vi "GlobalVariables.vi"() -> ()   [LabVIEW 2020]
panel:
  in  "Tab Control":T1(tab)
  in  "Ch4 LJ pin":string
  in  "LED Green pin":string
  in  "LED Red pin":string
  in  "Ch3 LJ pin":string
  in  "Ch2 LJ pin":string
  in  "Ch1 LJ pin":string
  out "TCP connected?":bool
  in  "LastUseiRF":T2
  in  "DeconChan Temp":T3(radio)=enum."Ch1"
  in  "SysCaliData":T4
  in  "BG4":dbl[](array[numeric])
  in  "BG3":dbl[](array[numeric])
  in  "BG2":dbl[](array[numeric])
  in  "BG1":dbl[](array[numeric])
  in  "DC Idx2":i32
  in  "DC Idx1":i32
  in  "BG Idx2":i32
  in  "BG Idx1":i32
  in  "Ch4GainLim(Log)":cluster{"GainMax":dbl, "GainMin":dbl}
  in  "Ch3GainLim(Log)":cluster{"GainMax":dbl, "GainMin":dbl}
  in  "Ch2GainLim(Log)":cluster{"GainMax":dbl, "GainMin":dbl}
  in  "Ch1GainLim(Log)":cluster{"GainMax":dbl, "GainMin":dbl}
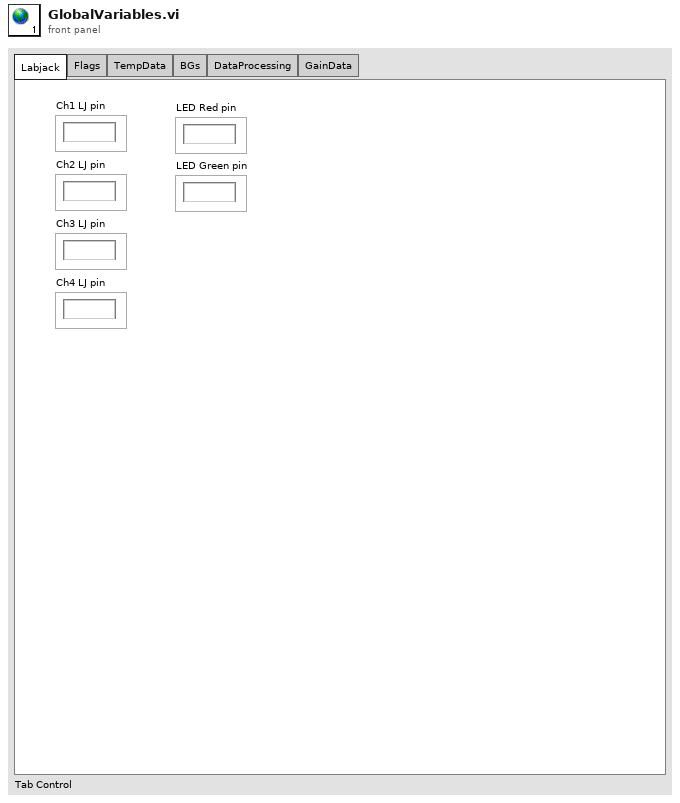
[diagram p1: front panel]
types:
  T1 = enum32{"Labjack", "Flags", "TempData", "BGs", "DataProcessing", "GainData"}
  T2 = cluster{"Ch1 iRF":dbl[], "Ch2 iRF":dbl[], "Ch3 iRF":dbl[], "Ch4 iRF":dbl[]}
  T3 = enum32{"No Selection", "Ch1", "Ch2", "Ch3", "Ch4"}
  T4 = cluster{"Ch1 WF":dbl[], "Ch2 WF":dbl[], "Ch3 WF":dbl[], "Ch4 WF":dbl[], "V1":dbl, "V2":dbl, "V3":dbl, "V4":dbl}
diagram:
